vi "Center Object.vi"(8 "error in":errorcluster, 9 "Rectangle":T1, 10 "Scrollbar Visible?":bool, 11 "Dialog in":refnum<class "Dialog.lvclass">) -> (0 "error out":errorcluster, 3 "Dialog.lvclass out":refnum<class "Dialog.lvclass">)   [LabVIEW 2012, in "Dialog.lvlib" / "Dialog.lvclass"]
uses:
  Dialog.lvclass
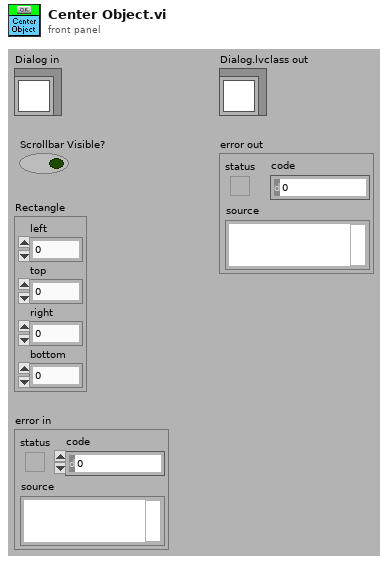
[diagram p1: front panel]
types:
  T1 = cluster{"left":i16, "top":i16, "right":i16, "bottom":i16}
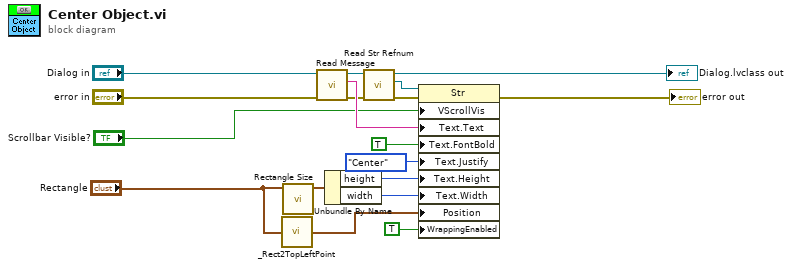
[diagram p0: block diagram]
diagram:
  n1 = call "_Rect2TopLeftPoint.vi"("bounds"="Rectangle") -> ("TopLeft point"=w16:cluster{"x":i32, "y":i32})  [unwired: 4 out]
  n2 = call "Rectangle Size.vi"("Rectangle"="Rectangle") -> ("Rect Size"=w15:cluster{"width":i32, "height":i32})  [unwired: 10 out]
  n3 = call-dynamic "Read Message.vi"("error in (no error)"="error in", "Dialog in"="Dialog in") -> ("error out"=w6:errorcluster, "Message"=w10:string, "Dialog out"=w7:refnum<class "Dialog.lvclass">)  [unwired: 7 out]
  n4 = Unbundle By Name(w15) -> ("height"=w12:i32, "width"=w13:i32)
  n5 = call-dynamic "Read Str Refnum.vi"("error in (no error)"=w6, "Dialog.lvclass in"=w7) -> ("error out"=w11:errorcluster, "Str Refnum"=w5:refnum<vi>, "Dialog.lvclass out"=→"Dialog.lvclass out":refnum<class "Dialog.lvclass">)  [unwired: 7 out]
  n6 = property class="Str"(reference=w5, error in=w11, "VScrollVis"="Scrollbar Visible?", "Text.Text"=w10, "Text.FontBold"=TRUE ("Size to Text?"), "Text.Justify"=enum16{"Left", "Center", "Right"}."Center" ("Justification"), "Text.Height"=w12, "Text.Width"=w13, "Position"=w16, "WrappingEnabled"=TRUE ("Enable Wrapping")) -> (error out=→"error out":errorcluster)  [unwired: 1 out]
